vi "Windows Media Player_LV2012_NI Verified.vi"() -> ()   [LabVIEW 2012]
doc: "This example VI opens Windows Media Player on your computer and plays a selected file."
panel:
  in  "Windows Media Player":refnum<k7>(container)
  # "Overview: This example VI opens Windows Media Player on your computer and plays a selected file.\nRequirements: LabVIEW 2012 (or compatible)\nInstructions:\nRun the VI"
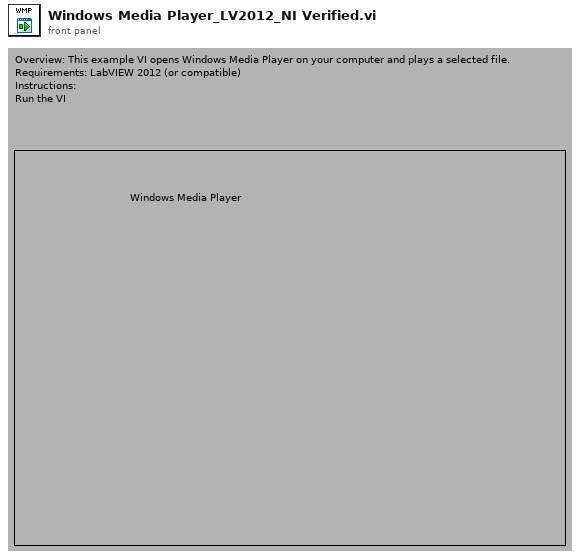
[diagram p1: front panel]
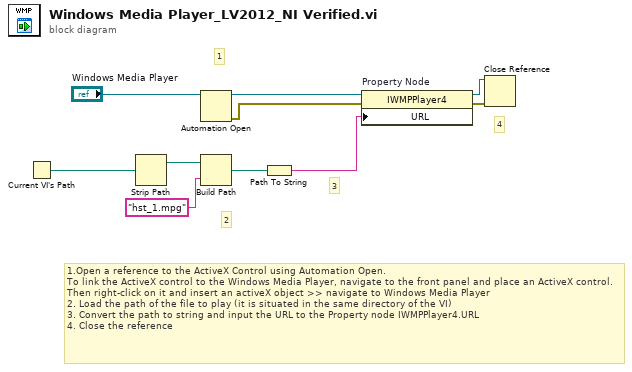
[diagram p0: block diagram]
diagram:
  # "1.Open a reference to the ActiveX Control using Automation Open. \nTo link the ActiveX control to the Windows Media Player, navigate to the front panel and place an ActiveX control. Then right-click on it and insert an activeX object >> navigate to Windows Media Player\n2. Load the path of the file to play (it is situated in the same directory of the VI)\n3. Convert the path to string and input the URL to the Property node IWMPPlayer4.URL\n4. Close the reference"
  # "4"
  # "3"
  # "2"
  # "1"
  n1 = Current VI's Path() -> (path=w5:path)
  n2 = Strip Path(path=w5) -> (stripped path=w4:path)  [unwired: 1 out]
  n3 = Automation Open(Automation Refnum="Windows Media Player") -> (Automation Refnum=w10:refnum<k7>, error out=w1:errorcluster)  [unwired: 1 in, 2 out]
  n4 = Build Path(base path=w4, name or relative path="hst_1.mpg") -> (appended path=w2:path)
  n5 = Path To String(path=w2) -> (string=w6:string)
  n6 = property on="Property Node" class="IWMPPlayer4"(reference=w10, error in=w1, "URL"=w6) -> (reference out=w8:refnum<k7>, error out=w7:errorcluster)
  n7 = Close Reference(reference=w8, error in (no error)=w7) -> ()  [unwired: 1 out]
